vi "Parse Named Entry.vi"(7 "SpreadsheetDocument in":refnum<k24>, 8 "error in":errorcluster, 9 "Cells":variant, 10 "Named Range":string, 11 "<JSON>":string="{}") -> (0 "error out":errorcluster, 3 "<JSON> out":string)   [LabVIEW 2019, in "Config from Excel Table.lvclass"]
uses:
  Config from Excel Table.lvclass
  Config from Excel Table.lvclass/Config from Excel Table.ctl
  3d530874-43db-4d28-b45c-a44206ee6d76.vi
  <vilib>/JDP Science/JSONtext/JSONtext.lvlib
  <vilib>/Peter/Open Xml/Source/Open Xml.lvlib
  <vilib>/Peter/Open Xml/Source/DocumentFormat.OpenXml.dll
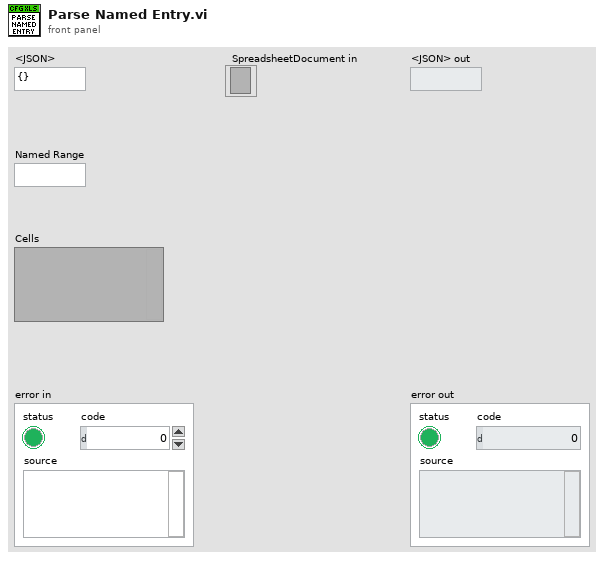
[diagram p1: front panel]
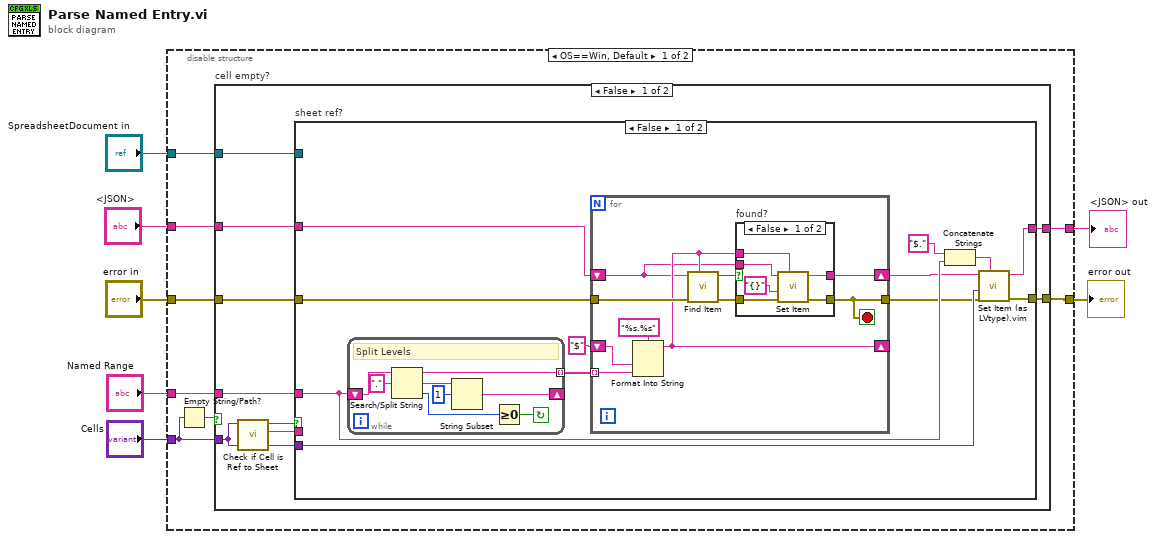
[diagram p0: block diagram]
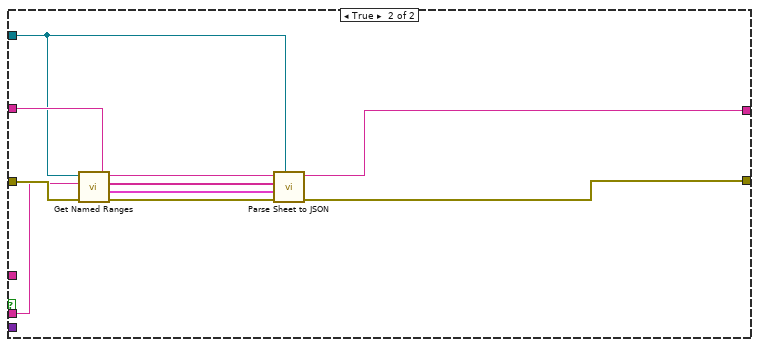
[diagram p3: hidden frame]
diagram:
  n1 = disable-structure shown="OS==Win, Default" {
    disable-tunnel: "Named Range" -> [w15 _]
    disable-tunnel: "<JSON>" -> [w14 _]
    disable-tunnel: "error in" -> [w13 w74]
    disable-tunnel: "SpreadsheetDocument in" -> [w12 _]
    disable-tunnel: [w11 _] -> w3
    disable-tunnel: [w10 w74] -> w2
    disable-tunnel: "Cells" -> [w8 _]
    frame condition #0 (active) {
      n2 = Empty String/Path?(string/path=w8) -> (empty?=w9:bool)
      n3 = case "cell empty?" shown="False" w9 {
        tunnel: w13 -> [w24 w73]
        tunnel: w12 -> [w23 _]
        tunnel: w8 -> [w20 _]
        tunnel: w14 -> [w19 w72]
        tunnel: w15 -> [w18 _]
        tunnel: [w17 w73] -> w10
        tunnel: [w16 w72] -> w11
        frame False {
          n4 = call "Check if Cell is Ref to Sheet.vi"("Value"=w20) -> ("Sheet Name"=w22:string, "Sheet Ref"=w21:bool)  [unwired: 9 in]
          n5 = case "sheet ref?" shown="False" w21 {
            tunnel: w24 -> [w28 w71]
            tunnel: w23 -> [_ w63]
            tunnel: w22 -> [_ w70]
            tunnel: [w32 w68] -> w17
            tunnel: w20 -> [w34 _]
            tunnel: w19 -> [w25 w64]
            tunnel: w18 -> [w31 _]
            tunnel: [w33 w67] -> w16
            frame False {
              n6 = while {
                shift-right: [w57] -> _
                shift-left: w31 -> [w56]
                tunnel: [w55] -> w30 mode=indexing
                stop <- w58 continue-if-true
                # "Split Levels"
                n7 = Search/Split String(string=w56, search string/char (-)=".") -> (substring before match=w55:string, match + rest of string=w59:string, offset of match=w61:i32)  [unwired: 1 in]
                n8 = String Subset(string=w59, offset (0)=1) -> (substring=w57:string)  [unwired: 1 in]
                n9 = Greater Or Equal To 0?(x=w61) -> (x >= 0?=w58:bool)
              }
              n10 = for {
                tunnel: w30 -> [w44] mode=indexing
                shift-right: [w39] -> _
                shift-left: "$" -> [w45]
                tunnel: w28 -> [w42]
                tunnel: [w41] -> w27
                shift-right: [w38] -> w26
                shift-left: w25 -> [w37]
                stop <- w41 stop-if-true
                n11 = Format Into String(format string="%s.%s", w45, w44) -> (resulting string=w39:string)  [unwired: 2 in, 1 out]
                n12 = call <vilib>:"Find Item.vi"("$Path or Item Name"=w39, "error in (no error)"=w42, "JSON"=w37) -> ("error out"=w43:errorcluster, "Found"=w40:bool)  [unwired: 5 in, 2 out]
                n13 = case "found?" shown="False" w40 {
                  tunnel: [w51 w53] -> w38
                  tunnel: [w50 w54] -> w41
                  tunnel: w43 -> [w49 w54]
                  tunnel: w39 -> [w48 _]
                  tunnel: w37 -> [w47 w53]
                  frame False {
                    n14 = call <vilib>:"Set Item.vi"("$Path or Item Name"=w48, "error in (no error)"=w49, "JSON to Insert"="{}", "JSON"=w47) -> ("error out"=w50:errorcluster, "<JSON>"=w51:string)  [unwired: 4 in, 1 out]
                  }
                  frame True {
                  }
                }
              }
              n15 = Concatenate Strings("$." ("string"), w31) -> (w35:string)
              n16 = call "Set Item (as LVtype).vim"("$Path or Item Name"=w35, "error in (no error)"=w27, "Anything"=w34, "JSON"=w26) -> ("error out"=w32:errorcluster, "<JSON>"=w33:string)  [unwired: 4 in, 1 out]
            }
            frame True {
              n17 = call <vilib>:"Get Named Ranges.vi"("error in"=w71, "Sheet Name"=w70, "SpreadsheetDoc in"=w63) -> ("error out"=w69:errorcluster, "Cells"=w66:cluster{"Cells":variant[][]}[], "Range Names"=w65:string[])  [unwired: 5 in, 1 out]
              n18 = call "Parse Sheet to JSON.vi"("SpreadsheetDocument in"=w63, "error in"=w69, "Cells"=w66, "Named Ranges"=w65, "<JSON> in"=w64) -> ("error out"=w68:errorcluster, "<JSON> out"=w67:string)  [unwired: 5 in]
            }
          }
        }
        frame True {
        }
      }
    }
    frame condition #1 {
    }
  }
  "error out" <- w2
  "<JSON> out" <- w3
